vi "Insert Bundle by Name in Wrapper.vi"(8 "error in (no error)":errorcluster, 11 "VI in":refnum<vi>) -> (0 "error out":errorcluster, 1 "Named Bundler":refnum<vi>, 2 "Wrapper Refnum":refnum<vi>)   [LabVIEW 2021, in "Converter.lvlib"]
uses:
  Converter.lvlib
  Converter Reusables/Converter Reusables.lvlib
  Path Functions/Path Functions.lvlib
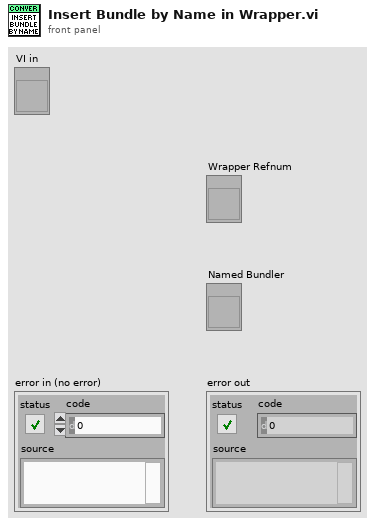
[diagram p1: front panel]
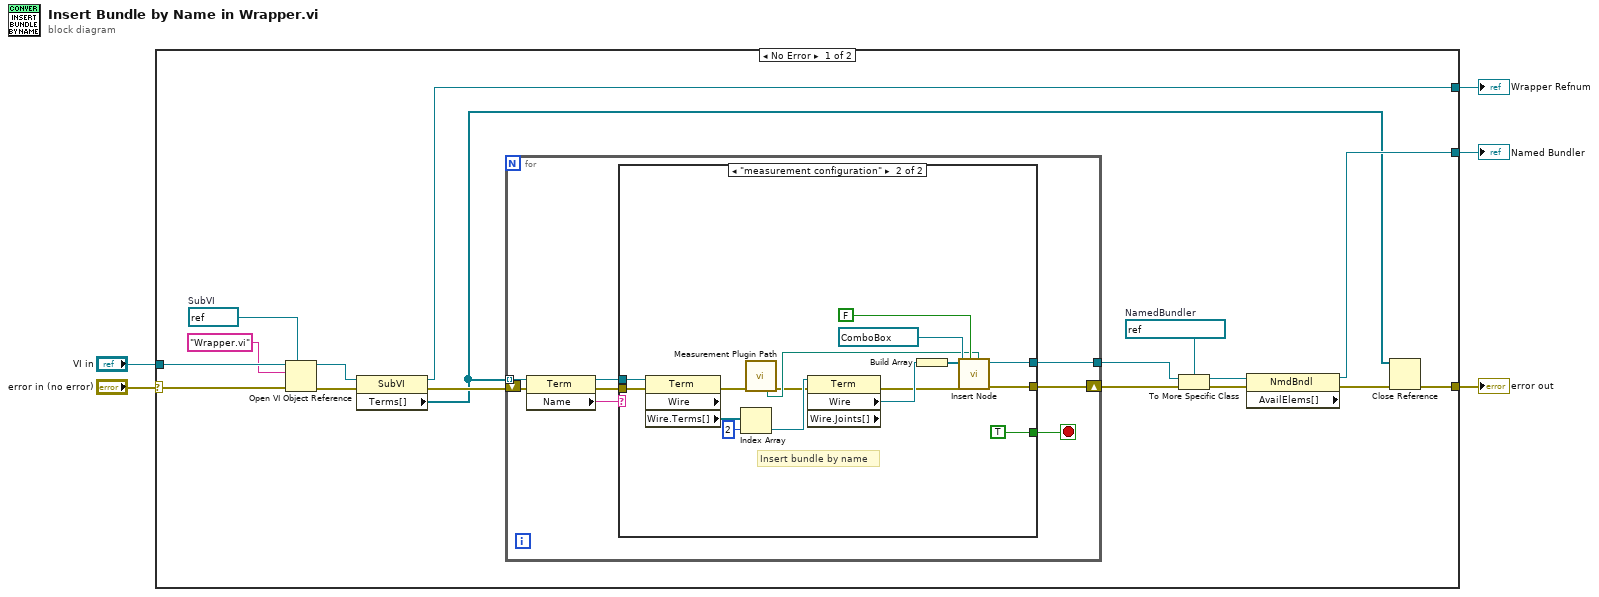
[diagram p0: block diagram]
diagram:
  n1 = case shown="No Error" "error in (no error)" {
    selector: "error in (no error)" -> [w19 w48]
    tunnel: "VI in" -> [w18 _]
    tunnel: [w13 _] -> w3
    tunnel: [w12 _] -> w2
    tunnel: [w11 w48] -> w1
    frame No Error {
      w22 = refnum<vi> refnum  # NamedBundler
      w20 = refnum<vi> refnum  # SubVI
      n2 = Open VI Object Reference(7:w20, 8:w19, 10:"Wrapper.vi" ("name/order"), 11:w18) -> (0:w15:errorcluster, 3:w17:refnum<vi>)
      n3 = property class="SubVI"(reference=w17, error in=w15) -> (reference out=w13:refnum<vi>, error out=w16:errorcluster, "Terms[]"=w10:refnum<vi>[])
      n4 = for {
        tunnel: w10 -> [w30] mode=indexing
        tunnel: [w24] -> w21
        shift-right: [w25] -> w7
        shift-left: w16 -> [w27]
        stop <- w23 stop-if-true
        n5 = property class="Term"(reference=w30, error in=w27) -> (reference out=w29:refnum<vi>, error out=w26:errorcluster, "Name"=w28:string)
        n6 = case shown="\"measurement configuration\"" w28 {
          tunnel: w29 -> [_ w43]
          tunnel: w26 -> [w31 w47]
          tunnel: [w31 w46] -> w25
          tunnel: [_ w45] -> w24
          tunnel: [_ TRUE] -> w23
          frame Default {
          }
          frame "measurement configuration" {
            # "Insert bundle by name"
            n7 = property class="Term" props=["Wire", "Wire", "Terms[]"](reference=w43, error in=w47) -> (error out=w33:errorcluster, "Wire.Terms[]"=w38:refnum<vi>[])  [unwired: 2 out]
            n8 = Index Array(array=w38, index=2) -> (element=w37:refnum<vi>)
            n9 = call "Measurement Plugin Path.vi"("error in (no error)"=w33) -> ("Logic VI Path"=w34:path, "error out"=w32:errorcluster)  [unwired: 2 in, 11 out]
            n10 = property class="Term" props=["Wire", "Wire", "Joints[]"](reference=w37, error in=w32) -> (error out=w35:errorcluster, "Wire"=w42:refnum<vi>)  [unwired: 2 out]
            n11 = Build Array(w42) -> (w39:refnum<vi>[])
            n12 = call "Insert Node.vi"("Path to LabVIEW File"=w34, "Shift Pressed?"=FALSE, "error in (no error)"=w35, "QD Combo Box Ref"=refnum<vi> refnum, "Selection List[]"=w39) -> ("error out"=w46:errorcluster, "element"=w45:refnum<vi>)  [unwired: 4 in, 1 out]
          }
        }
      }
      n13 = To More Specific Class(target class=w22, reference=w21, error in=w7) -> (specific class reference=w9:refnum<vi>, error out=w8:errorcluster)
      n14 = property class="NmdBndl" props=["AvailElems[]"](reference=w9, error in=w8) -> (reference out=w12:refnum<vi>, error out=w6:errorcluster)  [unwired: 1 out]
      n15 = Close Reference(reference=w10, error in (no error)=w6) -> (error out=w11:errorcluster)
    }
    frame Error {
    }
  }
  "error out" <- w1
  "Wrapper Refnum" <- w3
  "Named Bundler" <- w2
